vi "DMM data.vi"(0 "VISA resource name":refnum<visa-resource-name>, 1 "error in (no error)":errorcluster {"code" format="%.0x"}) -> (2 "Number of attempts":i32, 3 "Voltage":dbl, 4 "error out":errorcluster {"code" format="%.0x"})   [LabVIEW 2015]
uses:
  <instrlib>/Hameg DMM/Hameg DMM.lvlib
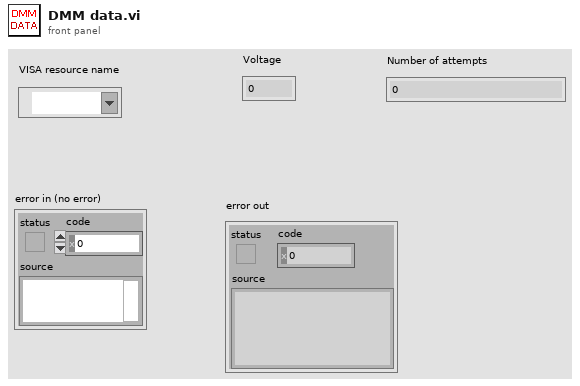
[diagram p1: front panel]
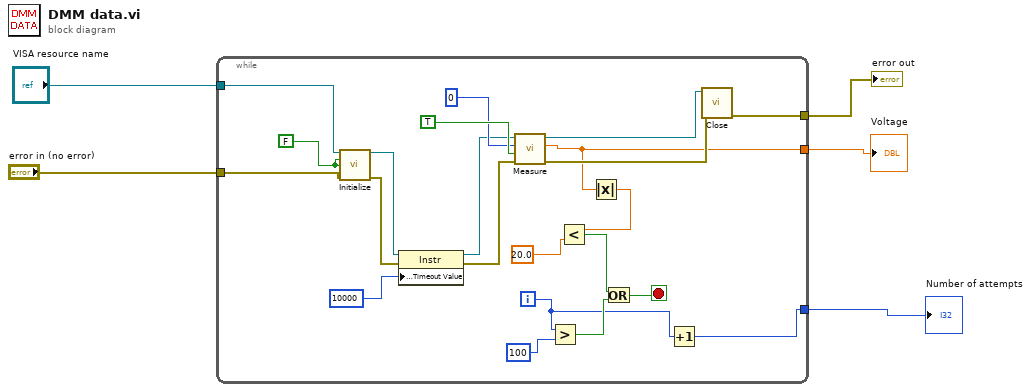
[diagram p0: block diagram]
diagram:
  n1 = while {
    tunnel: [w12] -> w5
    tunnel: "VISA resource name" -> [w23]
    tunnel: "error in (no error)" -> [w22]
    tunnel: [w16] -> w2
    tunnel: [w13] -> w1
    i -> [w17]
    stop <- w18 stop-if-true
    w24 = FALSE
    n2 = call <instrlib>:"Initialize.vi"("VISA resource name"=w23, "ID Query (T: Check)"=w24, "Reset (T: Reset)"=w24, "error in (no error)"=w22) -> ("VISA resource name out"=w9:refnum<visa-resource-name>, "error out"=w8:errorcluster)  [unwired: 10 in]
    n3 = property class="Instr"(reference=w9, error in=w8, "General Settings:Timeout Value"=u32 10000) -> (reference out=w7:refnum<visa-resource-name>, error out=w6:errorcluster)
    n4 = call <instrlib>:"Measure.vi"("error in (no error)"=w6, "Autorange (T: On)"=TRUE, "Function (0: DC Voltage)"=0, "VISA resource name"=w7) -> ("error out"=w15:errorcluster, "Measurement Value"=w12:dbl, "VISA resource name out"=w14:refnum<visa-resource-name>)  [unwired: 5 in]
    n5 = Greater?(x=w17, y=100) -> (0:w19:bool)
    n6 = Absolute Value(x=w12) -> (abs(x)=w11:dbl)
    n7 = Less?(x=w11, y=20.0) -> (x < y?=w20:bool)
    n8 = Or(x=w20, y=w19) -> (x .or. y?=w18:bool)
    n9 = Increment(x=w17) -> (x+1=w16:i32)
    n10 = call <instrlib>:"Close.vi"("error in (no error)"=w15, "VISA resource name"=w14) -> ("error out"=w13:errorcluster)  [unwired: 9 in]
  }
  "error out" <- w1
  "Voltage" <- w5
  "Number of attempts" <- w2
